vi "INIstring2DoubleArray.vi"(4 "String":string) -> (7 "Array":dbl[](array[numeric]))   [LabVIEW 2019]
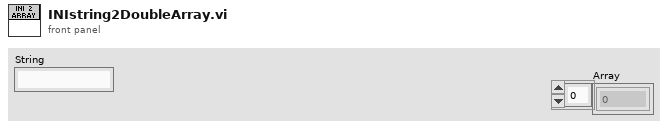
[diagram p1: front panel]
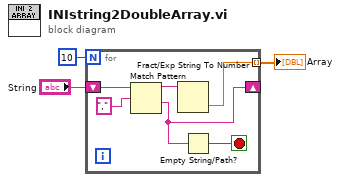
[diagram p0: block diagram]
diagram:
  n1 = for {
    N: 10 -> [_]
    shift-right: [w5] -> _
    shift-left: "String" -> [w9]
    tunnel: [w6] -> w2 mode=indexing
    stop <- w4 stop-if-true
    n2 = Match Pattern(string=w9, regular expression=",") -> (before substring=w8:string, after substring=w5:string)  [unwired: 1 in, 2 out]
    n3 = Fract/Exp String To Number(string=w8) -> (number=w6:dbl)  [unwired: 3 in, 1 out]
    n4 = Empty String/Path?(string/path=w5) -> (empty?=w4:bool)
  }
  "Array" <- w2
